vi "Open Log File.vi"(8 "error in (no error)":errorcluster, 11 "Datalogger Actor in":refnum<class "Datalogger Actor.lvclass">) -> (0 "error out":errorcluster, 3 "Datalogger Actor out":refnum<class "Datalogger Actor.lvclass">)   [LabVIEW 2018, in "Datalogger Actor.lvlib" / "Datalogger Actor.lvclass"]
uses:
  Datalogger Actor.lvclass
  Datalogger Actor.lvclass/Datalogger Actor.ctl
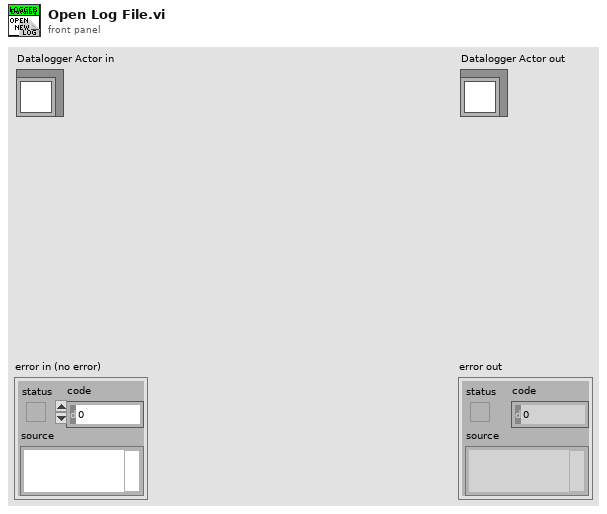
[diagram p1: front panel]
types:
  T1 = enum16{"open", "replace", "create", "open or create", "replace or create", "replace or create with confirmation"}
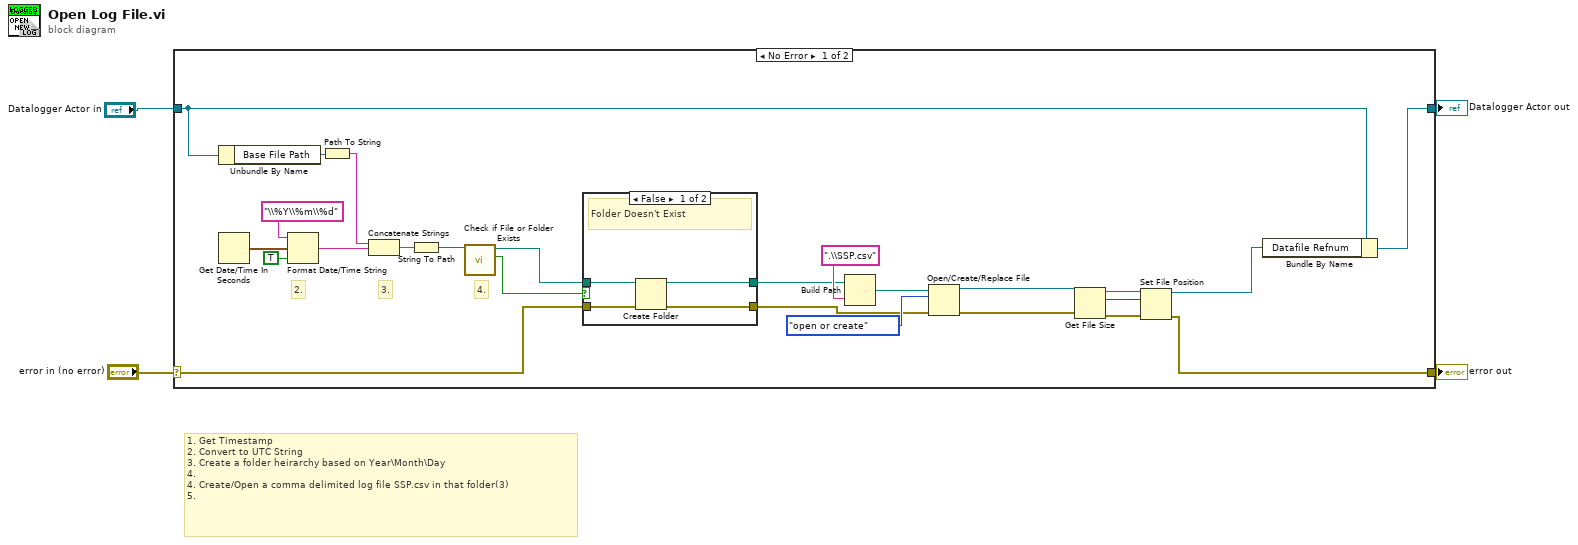
[diagram p0: block diagram]
diagram:
  # "1. Get Timestamp\n2. Convert to UTC String\n3. Create a folder heirarchy based on Year\\Month\\Day\n4. \n4. Create/Open a comma delimited log file SSP.csv in that folder(3)\n5."
  n1 = case shown="No Error" "error in (no error)" {
    selector: "error in (no error)" -> [w14 w37]
    tunnel: [w8 w37] -> w3
    tunnel: [w20 w36] -> w1
    tunnel: "Datalogger Actor in" -> [w21 w36]
    frame No Error {
      # "2."
      # "3."
      # "4."
      n2 = Unbundle By Name(w21) -> ("Base File Path"=w29:path)
      n3 = Get Date/Time In Seconds() -> (seconds since 1Jan1904=w25:timestamp)
      n4 = Format Date/Time String(time format string (%c)="\\%Y\\%m\\%d", seconds (now)=w25, UTC format=TRUE) -> (date/time string=w24:string)
      n5 = Path To String(path=w29) -> (string=w28:string)
      n6 = Concatenate Strings(w28, w24) -> (w27:string)
      n7 = String To Path(string=w27) -> (path=w7:path)
      n8 = call <vilib>:"Check if File or Folder Exists.vi"("path"=w7) -> ("file or folder exists?"=w6:bool, "dup path"=w5:path)  [unwired: 8 in, 1 out]
      n9 = case shown="False" w6 {
        tunnel: [w33 w34] -> w18
        tunnel: w14 -> [w32 w35]
        tunnel: [w31 w35] -> w13
        tunnel: w5 -> [w30 w34]
        frame False {
          # "Folder Doesn't Exist"
          n10 = Create Folder(path (use dialog)=w30, error in=w32) -> (created path=w33:path, error out=w31:errorcluster)  [unwired: 1 in, 1 out]
        }
        frame True {
          # "Folder Exists"
        }
      }
      n11 = Build Path(base path=w18, name or relative path=".\\SSP.csv" ("string")) -> (appended path=w17:path)
      n12 = Open/Create/Replace File(file path (use dialog)=w17, error in=w13, operation (0:open)=T1."open or create") -> (refnum out=w16:refnum<file>, error out=w15:errorcluster)  [unwired: 3 in, 1 out]
      n13 = Get File Size(file=w16, error in=w15) -> (refnum out=w10:refnum<file>, size (in bytes)=w11:i64, 0:w12:errorcluster)
      n14 = Set File Position(offset (in bytes) (0)=w11, refnum=w10, error in=w12) -> (refnum out=w9:refnum<file>, error out=w8:errorcluster)  [unwired: 1 in]
      n15 = Bundle By Name(cluster=w21, "Datafile Refnum"=w9) -> (w20:refnum<class "Datalogger Actor.lvclass">)
    }
    frame Error {
    }
  }
  "error out" <- w3
  "Datalogger Actor out" <- w1
